vi "EQ_parameters_Edit.vi"(6 "EQ parameters in":T1={"Timeout ITEST sweep"=6, "Number pulses ITEST"=5, "TOT"=40, "ADC target"=900, "Number pulses SSpeak sweep"=100, "Timeout SSpeak sweep"=110, "Timeout THLD sweep"=10, "Number triggers THLD sweep"=2, "First PIXEL"=0, "Last PIXEL"=0, "Sigma factor"=2, "DTP period for SSpeak sweep"=1, "Global THR for ITEST sweep"=38, "Pulse width"=0} {"Pulse width" items=["25 ns", "50 ns", "75 ns", "100 ns"]; "Global THR for ITEST sweep" step=1; "DTP period for SSpeak sweep" step=1; "Sigma factor" step=1; "Last PIXEL" max=99 step=1; "First PIXEL" max=99 step=1; "Number triggers THLD sweep" step=1; "Timeout THLD sweep" step=1; "Timeout SSpeak sweep" step=1; "Number pulses SSpeak sweep" step=1; "ADC target" step=1; "TOT" step=1; "Number pulses ITEST" step=1; "Timeout ITEST sweep" step=1}) -> (0 "EQ parameters (hex)":u32[](array[numeric])=[240000, 5, 1600, 900, 100, 4400000, 400000, 2, 0, 99, 2, 40000, 38, 0], 1 "EQ parameters Edited":T1={"Timeout ITEST sweep"=6, "Number pulses ITEST"=5, "TOT"=40, "ADC target"=900, "Number pulses SSpeak sweep"=100, "Timeout SSpeak sweep"=110, "Timeout THLD sweep"=10, "Number triggers THLD sweep"=2, "First PIXEL"=0, "Last PIXEL"=0, "Sigma factor"=2, "DTP period for SSpeak sweep"=1, "Global THR for ITEST sweep"=38, "Pulse width"=0} {"Pulse width" items=["25 ns", "50 ns", "75 ns", "100 ns"]; "Global THR for ITEST sweep" step=1; "DTP period for SSpeak sweep" step=1; "Sigma factor" step=1; "Last PIXEL" max=99 step=1; "First PIXEL" max=99 step=1; "Number triggers THLD sweep" step=1; "Timeout THLD sweep" step=1; "Timeout SSpeak sweep" step=1; "Number pulses SSpeak sweep" step=1; "ADC target" step=1; "TOT" step=1; "Number pulses ITEST" step=1; "Timeout ITEST sweep" step=1}, 2 "Number of pixels":u32=5 max=63 step=1)   [LabVIEW 2015, in "VIPM2.lvlib"]
uses:
  VIPM2.lvlib
panel:
  # "Edit EQ parameters meaning the restrictions"
  # "Transform to \"hex\" data"
  # "for autocalcul de timeout\nen altre subVI"
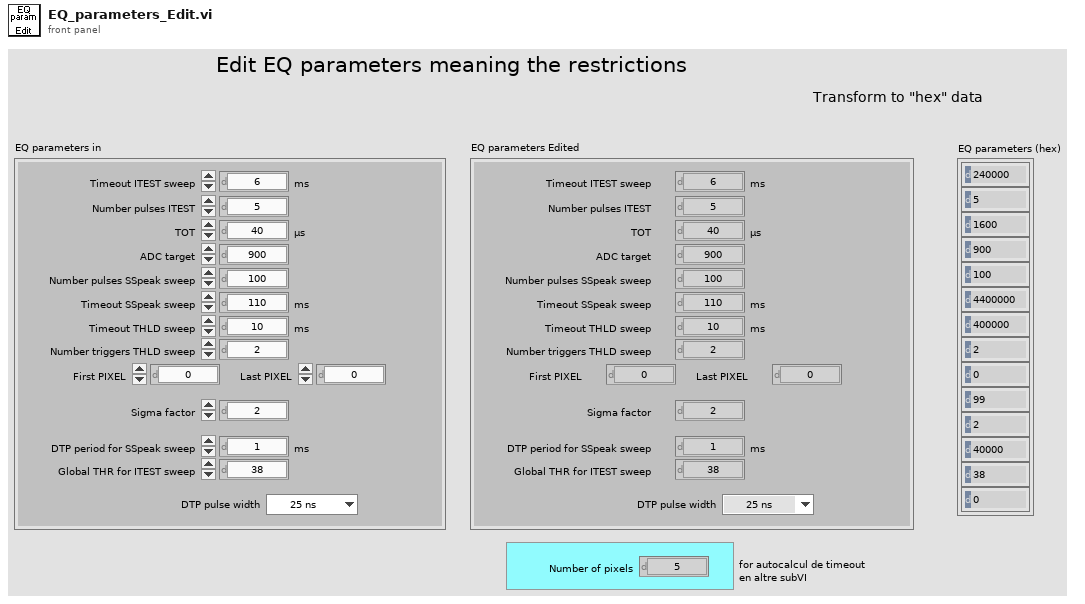
[diagram p1: front panel]
types:
  T1 = cluster{"Timeout ITEST sweep":u32, "Number pulses ITEST":u32, "TOT":u32, "ADC target":u32, "Number pulses SSpeak sweep":u32, "Timeout SSpeak sweep":u32, "Timeout THLD sweep":u32, "Number triggers THLD sweep":u32, "First PIXEL":u32, "Last PIXEL":u32, "Sigma factor":u32, "DTP period for SSpeak sweep":u32, "Global THR for ITEST sweep":u32, "Pulse width":u32}
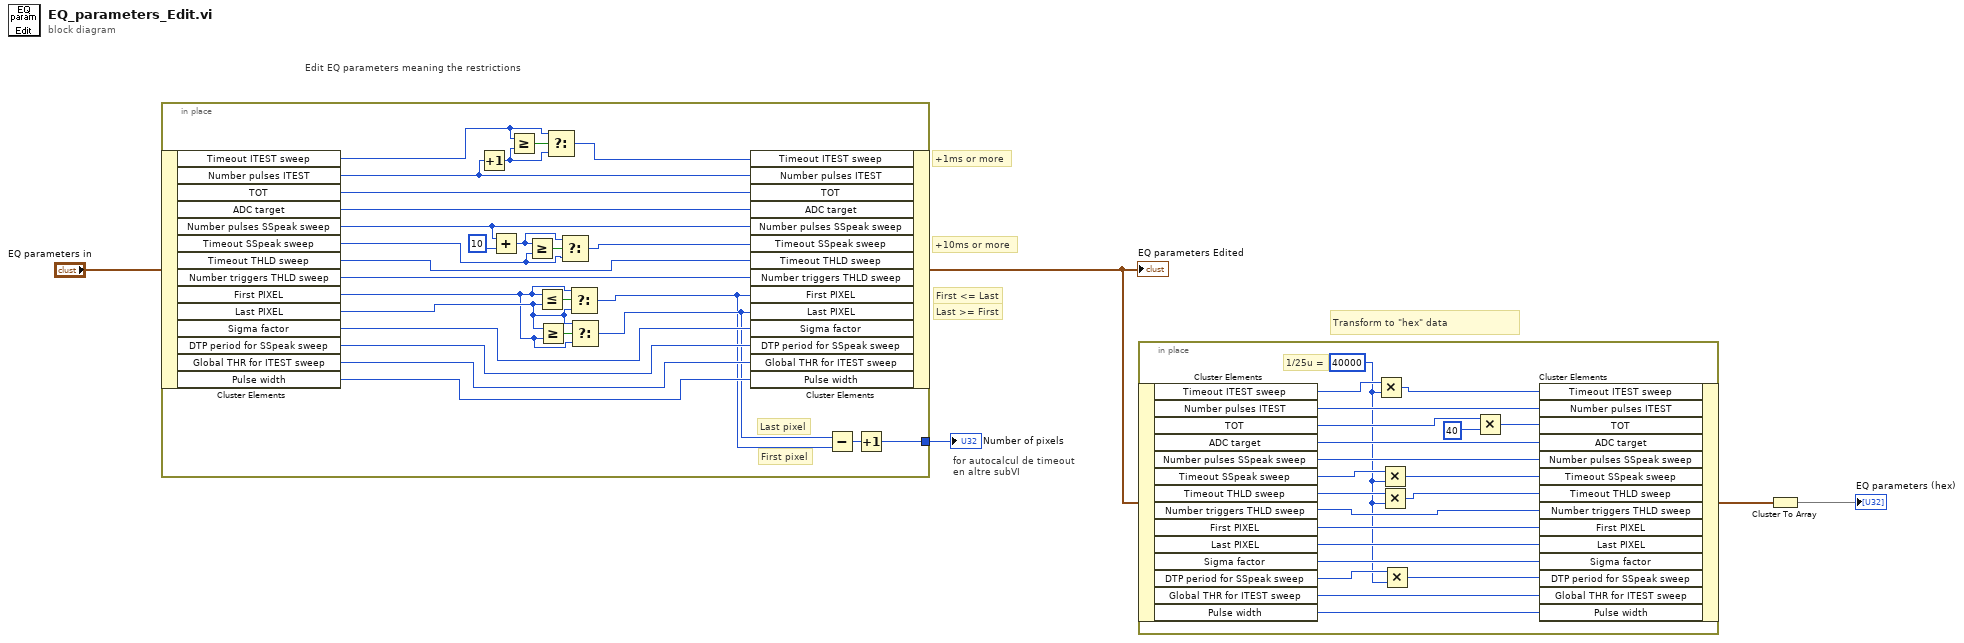
[diagram p0: block diagram]
diagram:
  # "Transform to \"hex\" data"
  # "Last >= First"
  # "First <= Last"
  # "+10ms or more"
  # "+1ms or more"
  # "for autocalcul de timeout\nen altre subVI"
  # "Edit EQ parameters meaning the restrictions"
  n1 = in-place {
    in-place-border: [w6] -> w5
    # "First pixel"
    # "Last pixel"
    n2 = in-place-cluster #1("EQ parameters in") -> ("Timeout ITEST sweep"=w30:u32, "Number pulses ITEST"=w32:u32, "TOT"=w27:u32, "ADC target"=w26:u32, "Number pulses SSpeak sweep"=w25:u32, "Timeout SSpeak sweep"=w21:u32, "Timeout THLD sweep"=w19:u32, "Number triggers THLD sweep"=w18:u32, "First PIXEL"=w14:u32, "Last PIXEL"=w15:u32, "Sigma factor"=w13:u32, "DTP period for SSpeak sweep"=w12:u32, "Global THR for ITEST sweep"=w11:u32, "Pulse width"=w10:u32)
    n3 = Increment(x=w32) -> (x+1=w29:u32)
    n4 = Add(x=w25, y=u32 10) -> (x+y=w22:u32)
    n5 = Greater Or Equal?(x=w30, y=w29) -> (x >= y?=w31:bool)
    n6 = Greater Or Equal?(x=w22, y=w21) -> (x >= y?=w23:bool)
    n7 = Less Or Equal?(x=w14, y=w15) -> (x <= y?=w17:bool)
    n8 = Greater Or Equal?(x=w15, y=w14) -> (x >= y?=w16:bool)
    n9 = Select(t=w30, s=w31, f=w29) -> (s? t:f=w28:u32)
    n10 = Select(t=w22, s=w23, f=w21) -> (s? t:f=w20:u32)
    n11 = Select(t=w14, s=w17, f=w15) -> (s? t:f=w8:u32)
    n12 = Select(t=w15, s=w16, f=w14) -> (s? t:f=w9:u32)
    n13 = in-place-cluster #1("Timeout ITEST sweep"=w28, "Number pulses ITEST"=w32, "TOT"=w27, "ADC target"=w26, "Number pulses SSpeak sweep"=w25, "Timeout SSpeak sweep"=w20, "Timeout THLD sweep"=w19, "Number triggers THLD sweep"=w18, "First PIXEL"=w8, "Last PIXEL"=w9, "Sigma factor"=w13, "DTP period for SSpeak sweep"=w12, "Global THR for ITEST sweep"=w11, "Pulse width"=w10) -> (w3:T1)
    n14 = Subtract(x=w9, y=w8) -> (x-y=w7:u32)
    n15 = Increment(x=w7) -> (x+1=w6:u32)
  }
  "Number of pixels" <- w5
  "EQ parameters Edited" <- w3
  n16 = in-place {
    w36 = u32 40000 ("y")
    # "1/25u ="
    n17 = in-place-cluster #2(w3) -> ("Timeout ITEST sweep"=w53:u32, "Number pulses ITEST"=w51:u32, "TOT"=w50:u32, "ADC target"=w48:u32, "Number pulses SSpeak sweep"=w47:u32, "Timeout SSpeak sweep"=w45:u32, "Timeout THLD sweep"=w43:u32, "Number triggers THLD sweep"=w41:u32, "First PIXEL"=w40:u32, "Last PIXEL"=w39:u32, "Sigma factor"=w38:u32, "DTP period for SSpeak sweep"=w37:u32, "Global THR for ITEST sweep"=w34:u32, "Pulse width"=w33:u32)
    n18 = Multiply(x=w53, y=w36) -> (x*y=w52:u32)
    n19 = Multiply(x=w45, y=w36) -> (x*y=w44:u32)
    n20 = Multiply(x=w43, y=w36) -> (x*y=w42:u32)
    n21 = Multiply(x=w37, y=w36) -> (x*y=w35:u32)
    n22 = Multiply(x=w50, y=u32 40) -> (x*y=w49:u32)
    n23 = in-place-cluster #2("Timeout ITEST sweep"=w52, "Number pulses ITEST"=w51, "TOT"=w49, "ADC target"=w48, "Number pulses SSpeak sweep"=w47, "Timeout SSpeak sweep"=w44, "Timeout THLD sweep"=w42, "Number triggers THLD sweep"=w41, "First PIXEL"=w40, "Last PIXEL"=w39, "Sigma factor"=w38, "DTP period for SSpeak sweep"=w35, "Global THR for ITEST sweep"=w34, "Pulse width"=w33) -> (w2:T1)
  }
  n24 = Cluster To Array(cluster=w2) -> (array=→"EQ parameters (hex)":u32[])
